vi "Get minimum separation within sphere.vi"(0 "Triangles to test":T2[](array[typedef]), 1 "Query triangles":T2[](array[typedef]), 2 "Octree for query triangles":T3[](array[typedef]), 3 "Sphere of interest":T1) -> (6 "Minimum separation vector\n(from all test triangles)":sgl[](array[numeric]), 7 "Minimum separation":sgl, 8 "Indices of possible triangles":i32[](array[numeric]))   [LabVIEW 2018]
doc: "This VI returns all the collision points between the test triangle and the query triangles, as well as the minimum separation vector and distance in the case of no collision."
uses:
  Typedefs/Triangle.ctl
  Typedefs/TreeNodeBox.ctl
  Typedefs/Quad.ctl
  Typedefs/Quadplane enum.ctl
  Typedefs/Sphere.ctl
  Globals/Trav_pos_global.vi
panel:
  # "PN 13/03/2015"
  # "Vertices"
  # "Edges"
  # "Unit normal"
  # "Edge unit normals"
  # "Vertices"
  # "Edges"
  # "Unit normal"
  # "Plane ident."
  # "Vertices"
  # "Edges"
  # "Unit normal"
  # "Plane ident."
  # "Vertices"
  # "Edges"
  # "Unit normal"
  # "Plane ident."
  # "Vertices"
  # "Edges"
  # "Unit normal"
  # "Plane ident."
  # "Vertices"
  # "Edges"
  # "Unit normal"
  # "Plane ident."
  # "Vertices"
  # "Edges"
  # "Unit normal"
  # "Plane ident."
  # "Vertices"
  # "Edges"
  # "Unit normal"
  # "Edge unit normals"
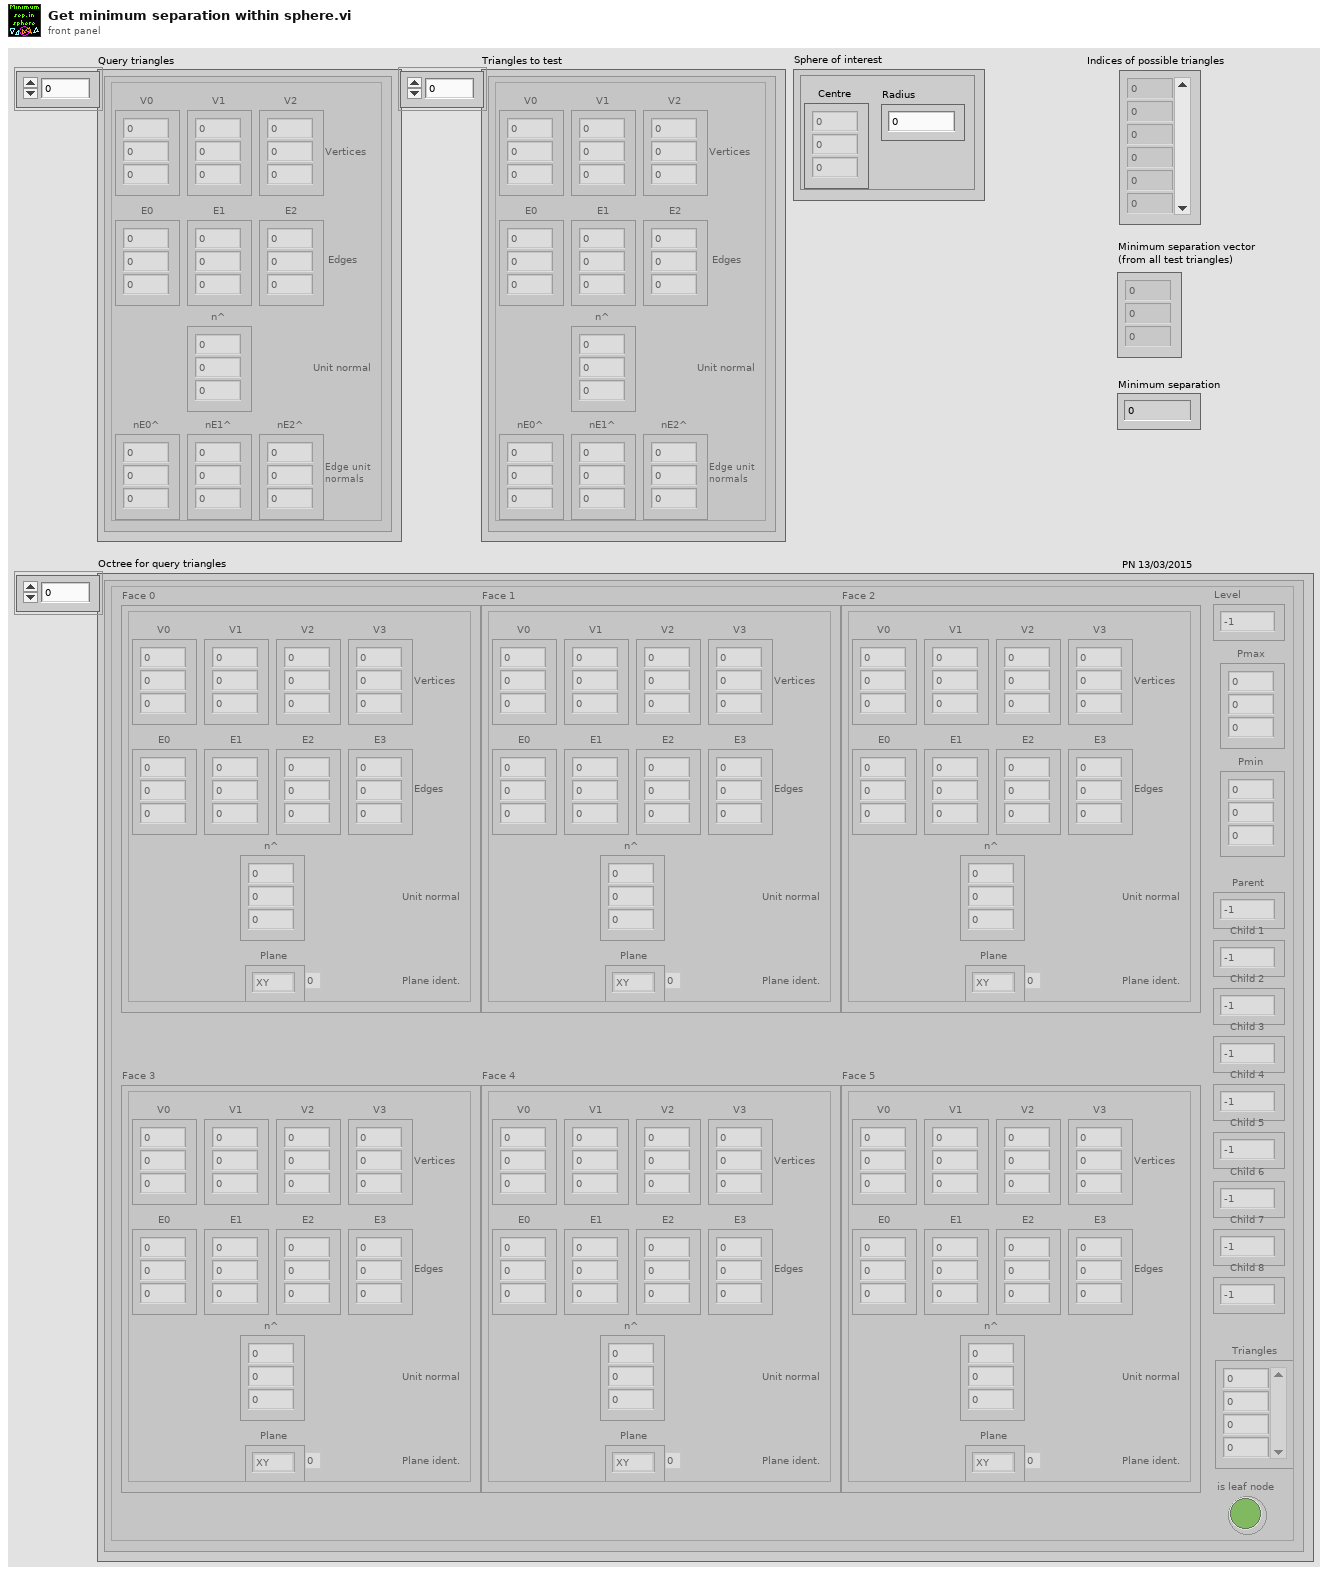
[diagram p1: front panel]
types:
  T1 = typedef "Sphere.ctl" = cluster{"Centre":sgl[], "Radius":sgl}
  T2 = typedef "Triangle.ctl" = cluster{"V0":sgl[], "V1":sgl[], "V2":sgl[], "E0":sgl[], "E1":sgl[], "E2":sgl[], "n^":sgl[], "nE0^":sgl[], "nE1^":sgl[], "nE2^":sgl[]}
  T3 = typedef "TreeNodeBox.ctl" = cluster{"Face 0":T4, "Face 1":T4, "Face 2":T4, "Face 3":T4, "Face 4":T4, "Face 5":T4, "Level":i32, "Pmax":sgl[], "Pmin":sgl[], "Parent":i32, "Child 1":i32, "Child 2":i32, "Child 3":i32, "Child 4":i32, "Child 5":i32, "Child 6":i32, "Child 7":i32, "Child 8":i32, "Triangles":i32[], "is leaf node":bool}
  T4 = typedef "Quad.ctl" = cluster{"V0":sgl[], "V1":sgl[], "V2":sgl[], "V3":sgl[], "E0":sgl[], "E1":sgl[], "E2":sgl[], "E3":sgl[], "n^":sgl[], "Plane":T5}
  T5 = typedef "Quadplane enum.ctl" = enum8{"XY", "XZ", "YZ", "-XY", "-XZ", "-YZ"}
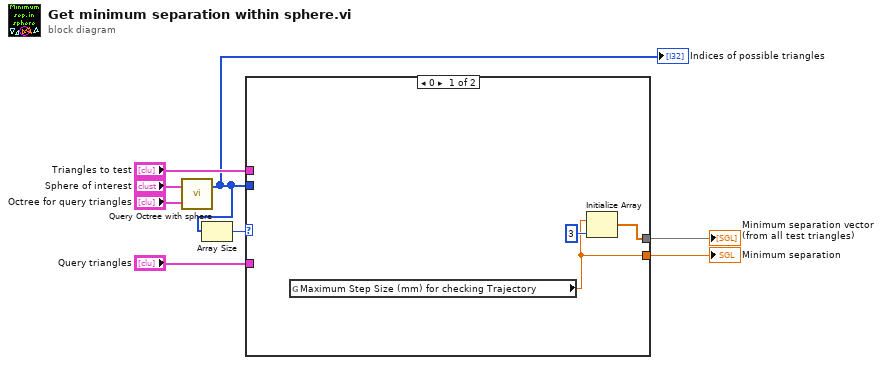
[diagram p0: block diagram]
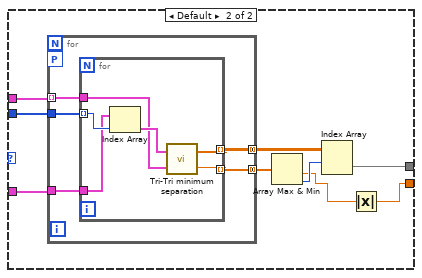
[diagram p2: hidden frame]
diagram:
  n1 = call "Query Octree with sphere.vi"("Octree node array"="Octree for query triangles", "Sphere"="Sphere of interest") -> ("Indices of possible triangles"=w2:i32[])  [unwired: 1 out]
  "Indices of possible triangles" <- w2
  n2 = Array Size(array=w2) -> (size(s)=w1:i32)
  n3 = case shown="0" w1 {
    tunnel: [w9 w12] -> w7
    tunnel: [w11 w19] -> w6
    tunnel: "Triangles to test" -> [_ w18]
    tunnel: w2 -> [_ w15]
    tunnel: "Query triangles" -> [_ w14]
    frame 0 {
      n4 = global read "Trav_pos_global.vi" "Maximum Step Size (mm) for checking Trajectory"() -> (w9:sgl)
      n5 = Initialize Array(w9, 3 ("dimension size")) -> (w11:sgl[])
    }
    frame Default {
      n6 = for {
        tunnel: [w25] -> w20 mode=concatenating
        tunnel: w18 -> [w24] mode=indexing
        tunnel: [w23] -> w16 mode=concatenating
        tunnel: w15 -> [w22]
        tunnel: w14 -> [w21]
        workers-P: _ -> [_]
        n7 = for {
          tunnel: w24 -> [w28]
          tunnel: w22 -> [w31] mode=indexing
          tunnel: [w30] -> w25 mode=indexing
          tunnel: [w27] -> w23 mode=indexing
          tunnel: w21 -> [w26]
          n8 = Index Array(array=w26, index=w31) -> (element=w29:T2)
          n9 = call "Tri-Tri minimum separation.vi"("Triangle 2"=w28, "Triangle 1"=w29) -> ("Minimum separation distance"=w30:sgl, "Minimum separation vector\nfrom triangle 2 to triange 1"=w27:sgl[])
        }
      }
      n10 = Array Max & Min(array=w20) -> (min value=w13:sgl, min index (indices)=w17:i32)  [unwired: 2 out]
      n11 = Index Array(array=w16, index (row)=w17) -> (element=w19:sgl[])  [unwired: 1 in]
      n12 = Absolute Value(x=w13) -> (abs(x)=w12:sgl)
    }
  }
  "Minimum separation" <- w7
  "Minimum separation vector\n(from all test triangles)" <- w6
